vi "Msg EnQ.vi"(9 "Msg":refnum<class "Msg.lvclass">, 10 "Msg Q":refnum<class "Msg Q.lvclass">, 11 "Msg EnQ in":refnum<class "Msg EnQ.lvclass">) -> (0 "error out":errorcluster)   [LabVIEW 2021, in "AAM.lvlib" / "Msg EnQ.lvclass"]
uses:
  Msg EnQ.lvclass
  Msg/Msg.lvclass
  Msg Q/Msg Q.lvclass
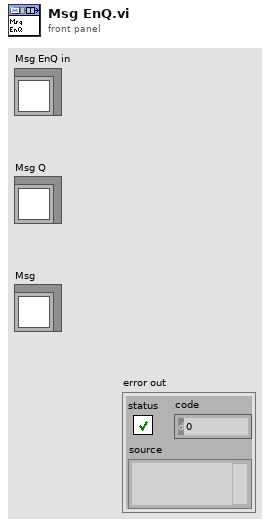
[diagram p1: front panel]
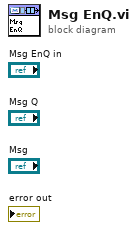
[diagram p0: block diagram]
diagram:
